vi "Add Library To Project.vi"(8 "error in":errorcluster, 9 "New Library Name":string, 10 "Library Path":path, 11 "Project ref":refnum<vi>) -> (0 "error out":errorcluster)   [LabVIEW 2020, in "MeasurementService Editor.lvlib"]
uses:
  MeasurementService Editor.lvlib
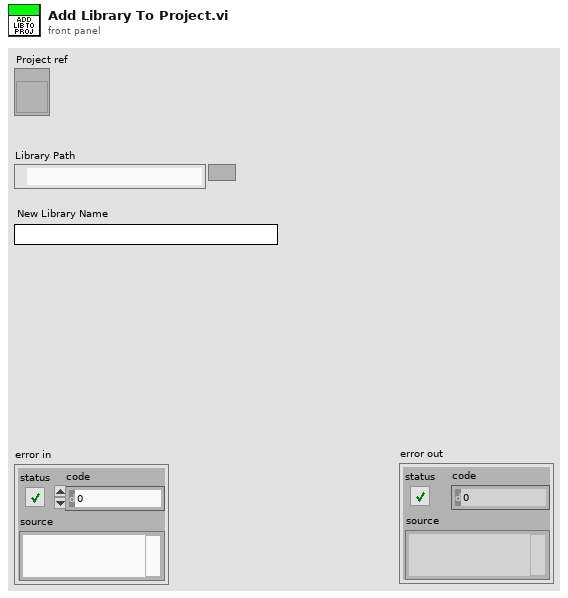
[diagram p1: front panel]
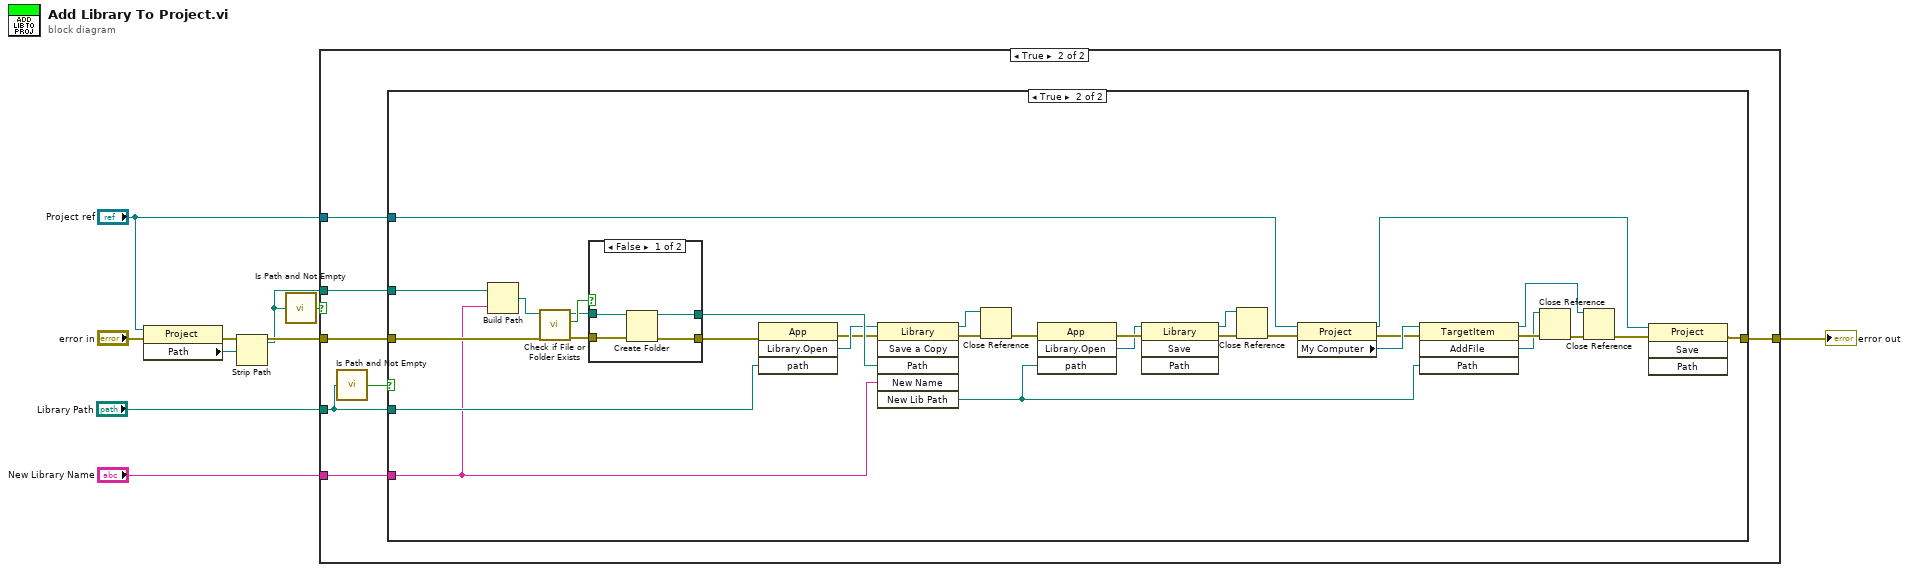
[diagram p0: block diagram]
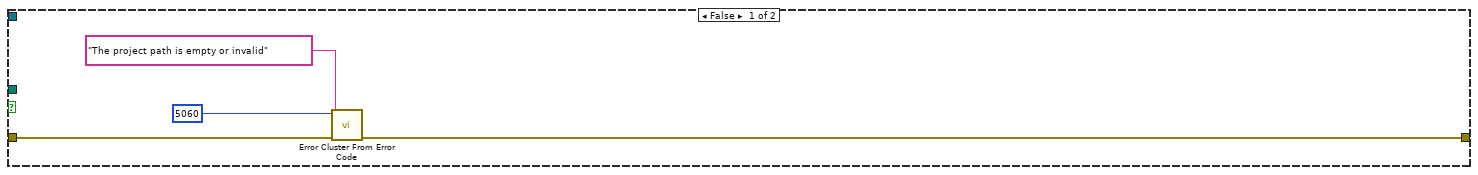
[diagram p2: hidden frame]
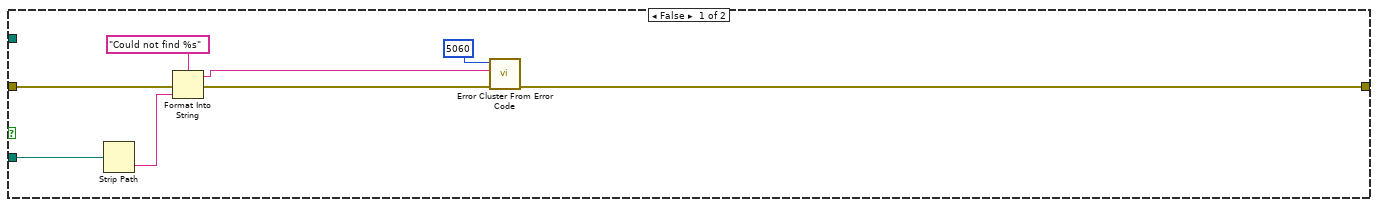
[diagram p3: hidden frame]
diagram:
  n1 = property class="Project"(reference="Project ref", error in="error in") -> (error out=w6:errorcluster, "Path"=w3:path)  [unwired: 1 out]
  n2 = Strip Path(path=w3) -> (stripped path=w2:path)  [unwired: 1 out]
  n3 = call <vilib>:"Is Path and Not Empty.vi"("path"=w2) -> ("Is Path and Not Empty?"=w9:bool)  [unwired: 4 in]
  n4 = case shown="True" w9 {
    tunnel: w6 -> [w13 w20]
    tunnel: [w12 w19] -> w8
    tunnel: "Library Path" -> [_ w17]
    tunnel: "New Library Name" -> [_ w16]
    tunnel: w2 -> [_ w15]
    tunnel: "Project ref" -> [_ w14]
    frame False {
      n5 = call <vilib>:"Error Cluster From Error Code.vi"("error in (no error)"=w13, "error message (\"\")"="The project path is empty or invalid" ("error message (\"\")"), "error code (0)"=5060) -> ("error out"=w12:errorcluster)  [unwired: 6 in]
    }
    frame True {
      n6 = call <vilib>:"Is Path and Not Empty.vi"("path"=w17) -> ("Is Path and Not Empty?"=w18:bool)  [unwired: 4 in]
      n7 = case shown="True" w18 {
        tunnel: w20 -> [w27 w59]
        tunnel: [w26 w57] -> w19
        tunnel: w17 -> [w23 w58]
        tunnel: w16 -> [_ w48]
        tunnel: w15 -> [_ w56]
        tunnel: w14 -> [_ w55]
        frame False {
          n8 = Strip Path(path=w23) -> (name=w24:string)  [unwired: 1 out]
          n9 = Format Into String(format string="Could not find %s", error in=w27, w24) -> (resulting string=w21:string, error out=w25:errorcluster)  [unwired: 1 in]
          n10 = call <vilib>:"Error Cluster From Error Code.vi"("error in (no error)"=w25, "error message (\"\")"=w21, "error code (0)"=5060) -> ("error out"=w26:errorcluster)  [unwired: 6 in]
        }
        frame True {
          n11 = Build Path(base path=w56, name or relative path=w48) -> (appended path=w54:path)
          n12 = call <vilib>:"Check if File or Folder Exists.vi"("error in (no error)"=w59, "path"=w54) -> ("error out"=w51:errorcluster, "file or folder exists?"=w53:bool, "dup path"=w52:path)  [unwired: 7 in]
          n13 = case shown="False" w53 {
            tunnel: w52 -> [w62 w65]
            tunnel: w51 -> [w63 w64]
            tunnel: [w61 w64] -> w50
            tunnel: [w60 w65] -> w49
            frame False {
              n14 = Create Folder(path (use dialog)=w62, error in=w63) -> (created path=w60:path, error out=w61:errorcluster)  [unwired: 1 in, 1 out]
            }
            frame True {
            }
          }
          n15 = invoke class="App" method="Library.Open"(error in=w50, "path"=w58) -> (error out=w33:errorcluster, "Open Library"=w47:refnum<vi>)  [unwired: 2 in, 2 out]
          n16 = invoke class="Library" method="Save a Copy"(reference=w47, error in=w33, "Path"=w49, "New Name"=w48) -> (reference out=w42:refnum<vi>, error out=w44:errorcluster, "New Lib Path"=w32:path)  [unwired: 2 in, 3 out]
          n17 = Close Reference(reference=w42, error in (no error)=w44) -> (error out=w43:errorcluster)
          n18 = invoke class="App" method="Library.Open"(error in=w43, "path"=w32) -> (error out=w41:errorcluster, "Open Library"=w40:refnum<vi>)  [unwired: 2 in, 2 out]
          n19 = invoke class="Library" method="Save"(reference=w40, error in=w41) -> (reference out=w38:refnum<vi>, error out=w39:errorcluster)  [unwired: 2 in, 2 out]
          n20 = Close Reference(reference=w38, error in (no error)=w39) -> (error out=w37:errorcluster)
          n21 = property class="Project"(reference=w55, error in=w37) -> (reference out=w34:refnum<vi>, error out=w45:errorcluster, "My Computer"=w46:refnum<vi>)
          n22 = invoke class="TargetItem" method="AddFile"(reference=w46, error in=w45, "Path"=w32) -> (reference out=w29:refnum<vi>, error out=w36:errorcluster, "AddFile"=w35:refnum<vi>)  [unwired: 1 in, 1 out]
          n23 = Close Reference(reference=w35, error in (no error)=w36) -> (error out=w31:errorcluster)
          n24 = Close Reference(reference=w29, error in (no error)=w31) -> (error out=w30:errorcluster)
          n25 = invoke class="Project" method="Save"(reference=w34, error in=w30) -> (error out=w57:errorcluster)  [unwired: 2 in, 3 out]
        }
      }
    }
  }
  "error out" <- w8
